vi "Butterfly_PullDown RCV_TTR_AWG.vi"(0 "Semiconductor Module Context":T2, 1 "RFPins":string[](array[string]), 2 "script name":string, 3 "R Thresholds":dbl[](array[numeric]), 4 "Capacitance":bool=TRUE, 5 "error in (no error)":errorcluster, 6 "VNAs Measurement Parameters":T1, 7 "Start_v":dbl=10.0 format="%#_13g", 8 "C_TH_Delta":dbl=2.0, 9 "Stop_v":dbl=41.0 format="%#_13g", 11 "Step_v":dbl=1.0) -> (14 "Semiconductor Module Context Out":T2, 19 "error out":errorcluster)   [LabVIEW 2013]
uses:
  <vilib>/NI_TestStand_SemiconductorModule/NI_TestStand_Semiconductor_Module.lvlibp/PinMap/General/SemiconductorModuleContext.ctl
  VNA/VNAs Measurement Parameters.ctl
  <instrlib>/niHSDIO/niHSDIO.llb/niHSDIO_ctl Trigger Script - trigID Values (Ring).ctl
  <instrlib>/niDCPower/nidcpower.llb/niDCPower Wait For Event - Event.ctl
  <vilib>/NI_TestStand_SemiconductorModule/NI_TestStand_Semiconductor_Module.lvlibp/PinMap/DC Power/PinsToNIDCPowerSessions.vi
  <vilib>/NI_TestStand_SemiconductorModule/NI_TestStand_Semiconductor_Module.lvlibp/PinMap/General/Publish/PublishDataDoubleFunctionalTest.vi
  <vilib>/NI_TestStand_SemiconductorModule/NI_TestStand_Semiconductor_Module.lvlibp/PinMap/General/Publish/PublishDataDouble2D.vi
  <vilib>/NI_TestStand_SemiconductorModule/NI_TestStand_Semiconductor_Module.lvlibp
  VNA/Pin Map API/VNA Custom Instrument.lvlib
panel:
  in  "current level":dbl=0.01 format="%_6p"
  out "VPIs 2":dbl[](array[numeric])
  out "VRLs 2":dbl[](array[numeric])
  out "S0 steps":dbl[](array[numeric]) format="%#_3g"
  out "S1 steps":dbl[](array[numeric]) format="%#_3g"
  out "S2 steps":dbl[](array[numeric]) format="%#_3g"
  out "S3 steps":dbl[](array[numeric]) format="%#_3g"
  out "appended array":dbl[][](array[numeric]) format="%#_3g"
  out "VPIs":dbl[][](array[numeric]) format="%#_3g"
  out "VRLs":dbl[][](array[numeric]) format="%#_3g"
  out "C_Free":dbl[](array[numeric])
  out "Full R Array":dbl[][][](array[numeric])
  out "step":i32
  out "sites and pins loop iter":i32
  out "BF values":dbl[](array[numeric])
  out "BF Names":string[](array[string])
  out "R Array":dbl[](array[numeric])
  out "BFSamples":i32
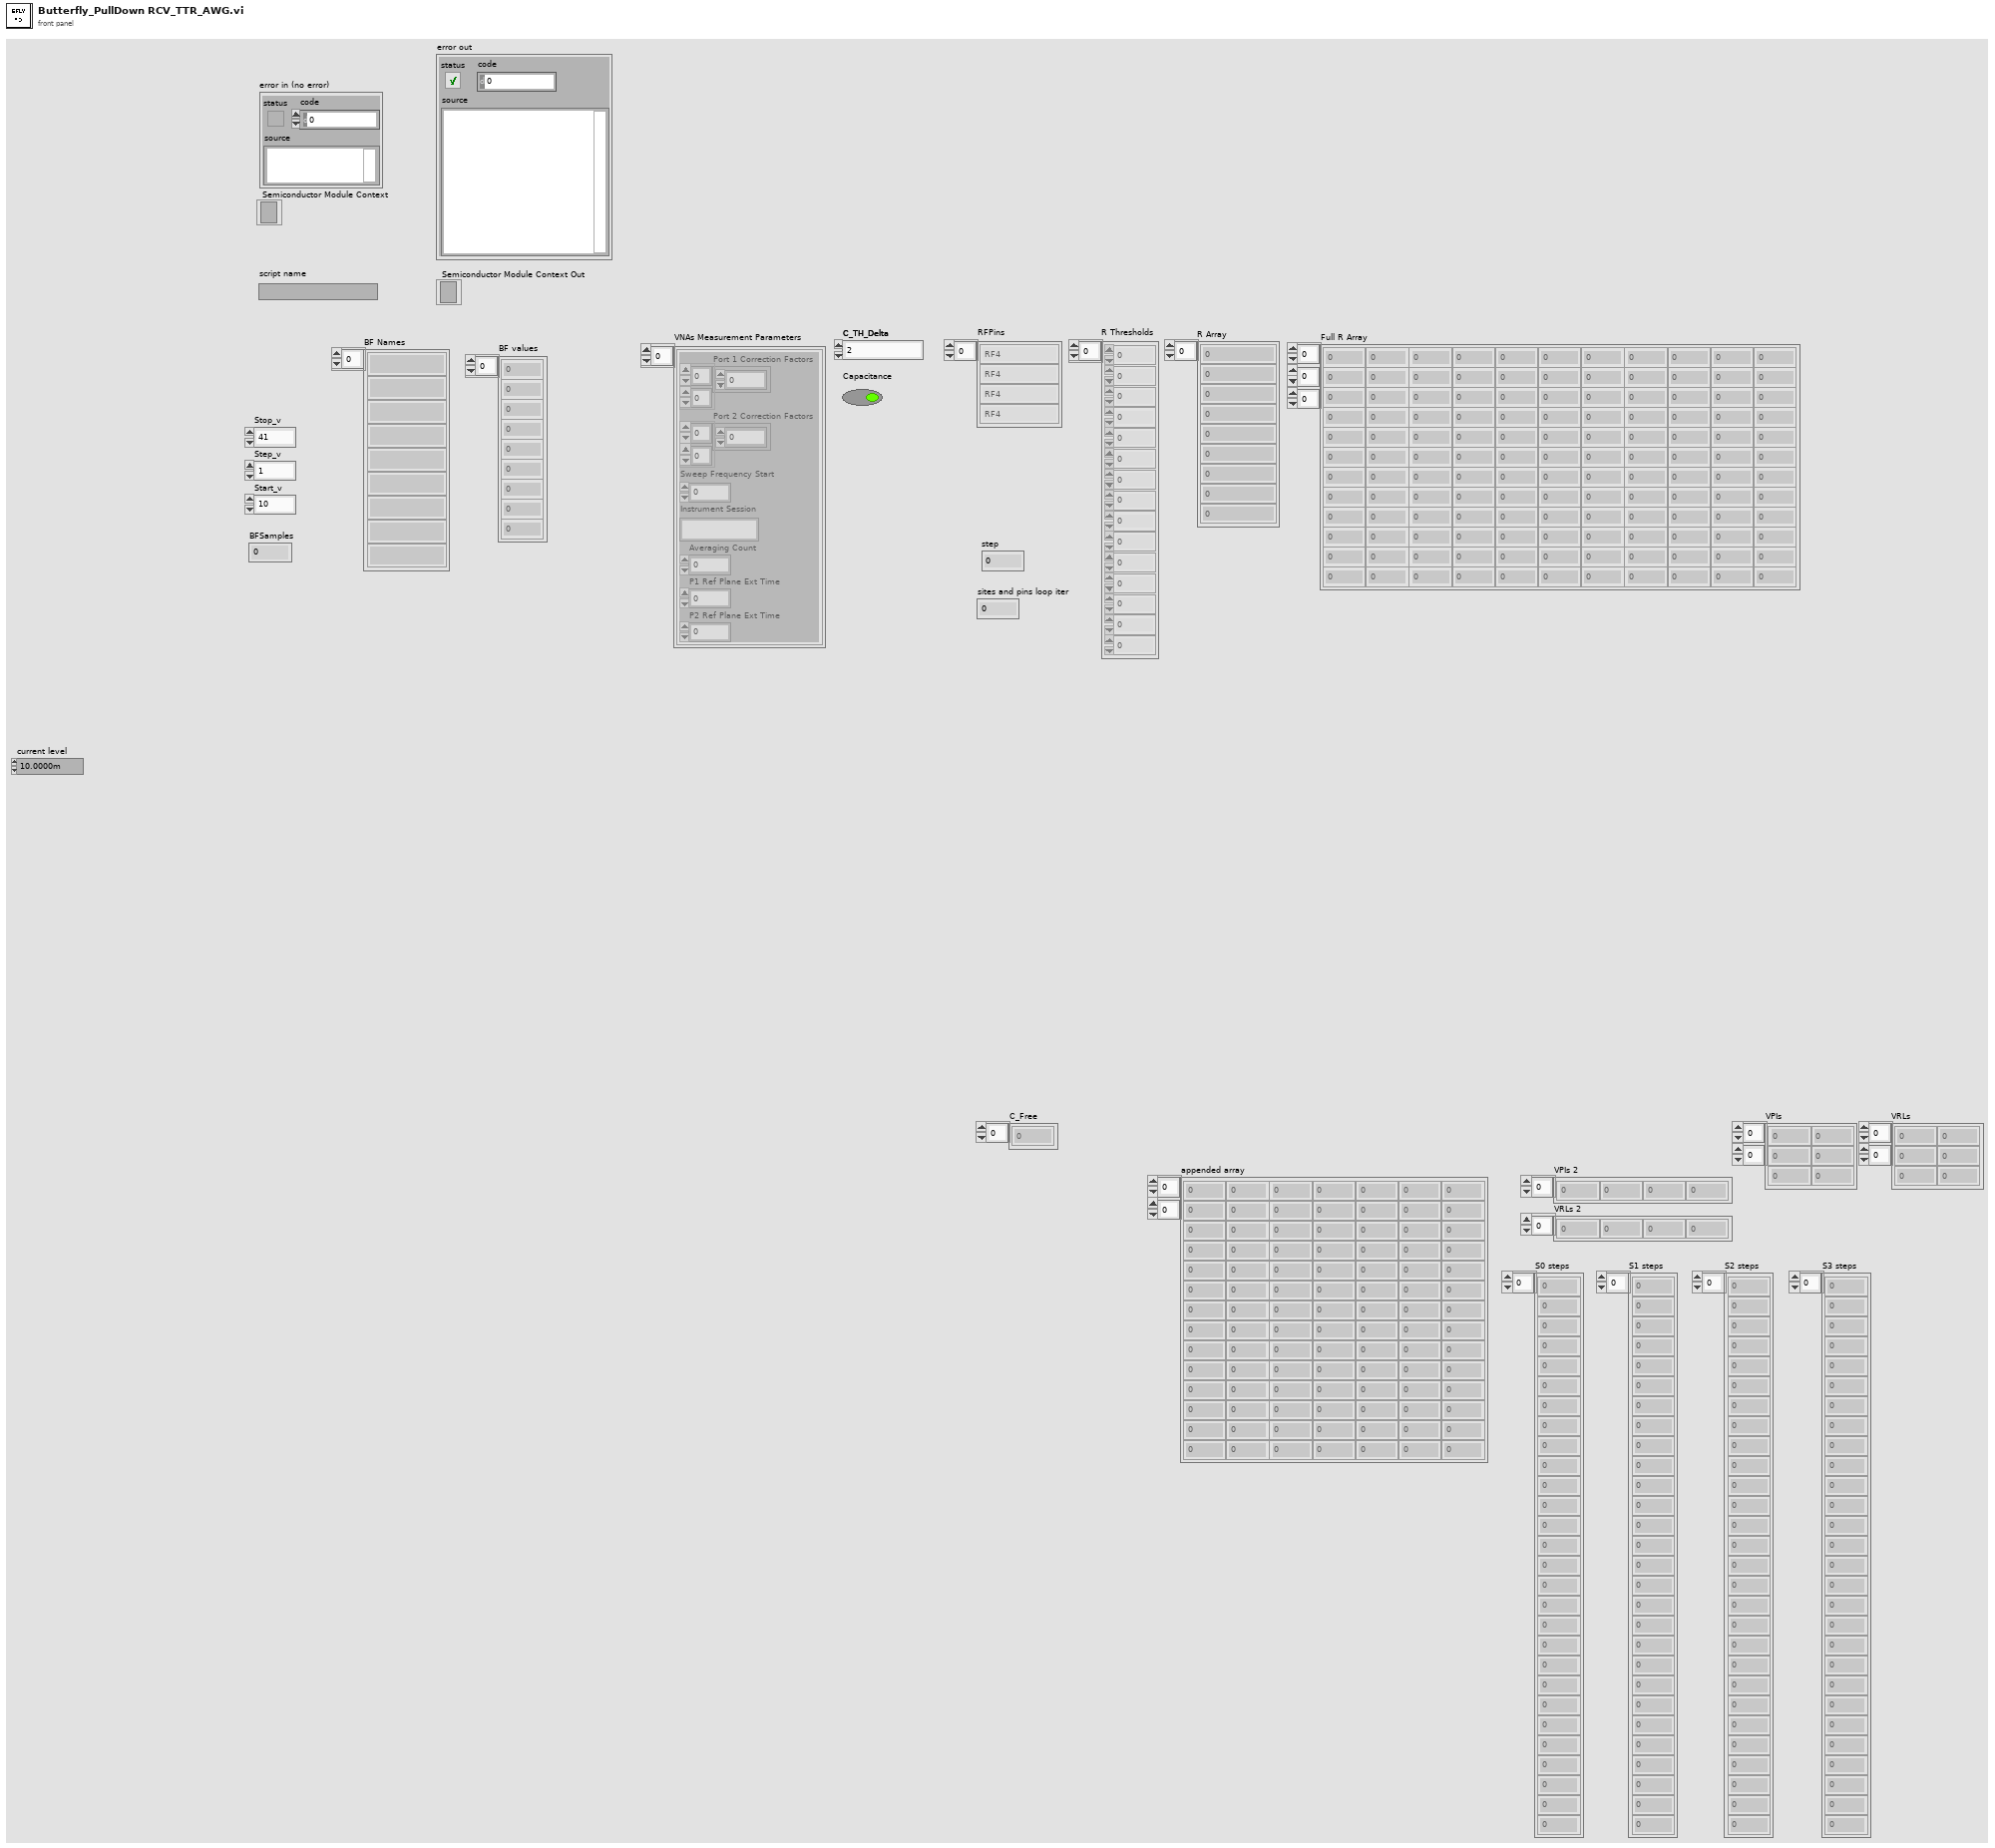
[diagram p1: front panel]
types:
  T1 = typedef "VNAs Measurement Parameters.ctl" = cluster{"Port 1 Correction Factors":cdb[][], "Port 2 Correction Factors":cdb[][], "Sweep Frequency Start":dbl, "Instrument Session":string, "Averaging Count":i32, "P1 Ref Plane Ext Time":dbl, "P2 Ref Plane Ext Time":dbl}[]
  T2 = typedef "NI_TestStand_Semiconductor_Module.lvlibp/SemiconductorModuleContext.ctl" = refnum<k7>
  T3 = typedef "niDCPower Wait For Event - Event.ctl" = i32
  T4 = typedef "niHSDIO_ctl Trigger Script - trigID Values (Ring).ctl" = string
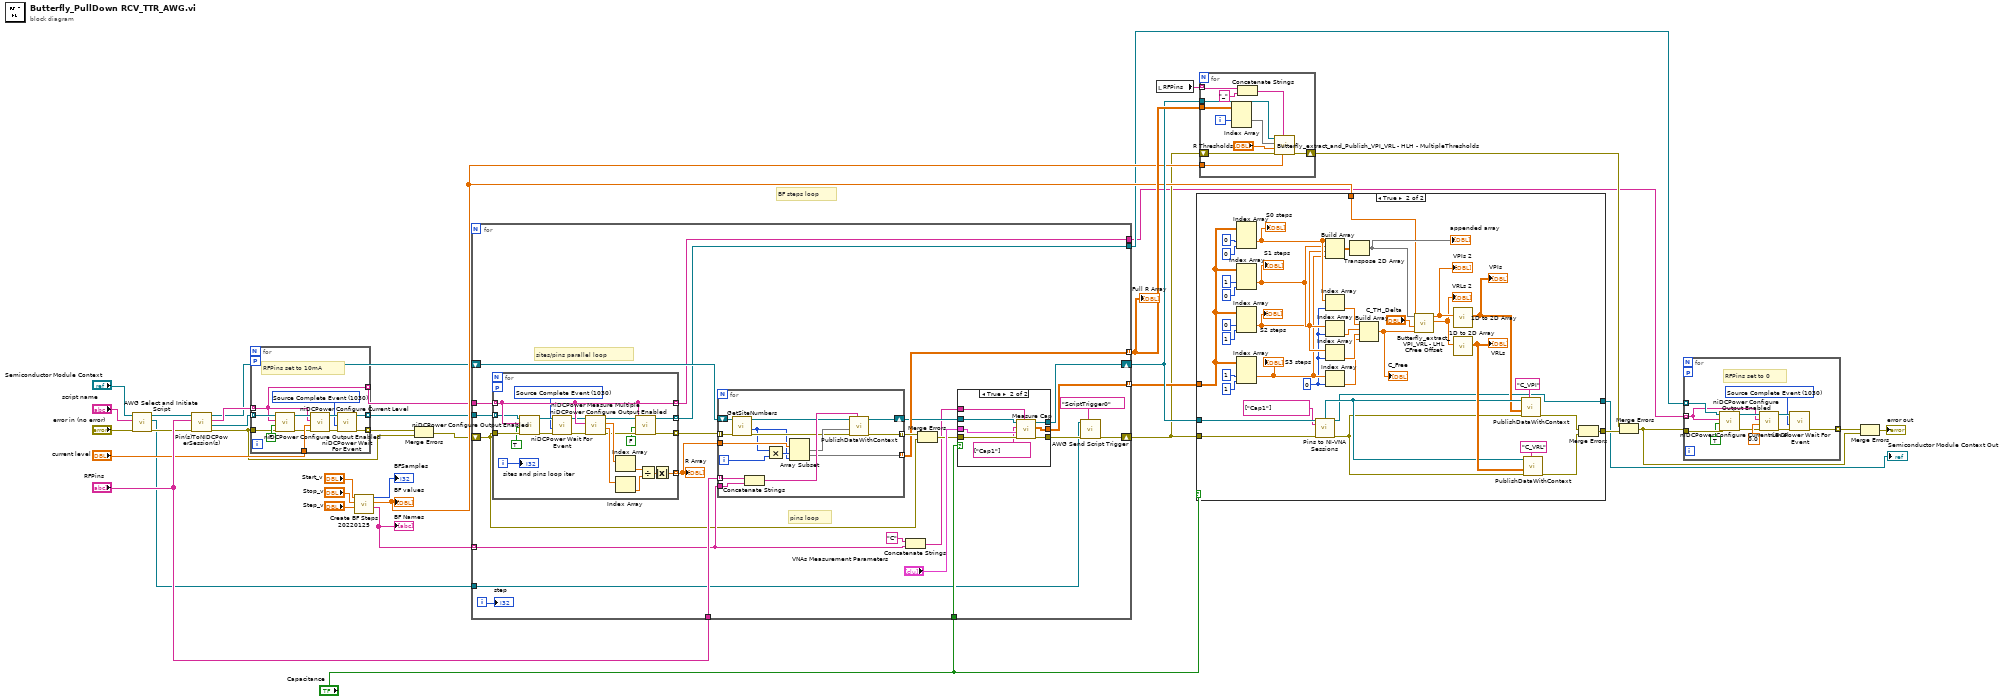
[diagram p0: block diagram]
diagram:
  # "BF steps loop"
  n1 = call "AWG Select and Initiate Script.vi"("error in (no error)"="error in (no error)", "script name"="script name", "Semiconductor Module Context"="Semiconductor Module Context") -> ("error out"=w6:errorcluster, "Sessions Out"=w1:refnum<k15>[], "Semiconductor Module Context Out"=w8:T2)  [unwired: 6 in]
  n2 = call-poly <vilib>:"Pin(s)ToNIDCPowerSession(s).vi"("error in (no error)"=w6, "Pins"="RFPins", "Semiconductor Module Context"=w8) -> ("error out"=w10:errorcluster, "Instrument Sessions"=w20:refnum<k15>[], "Channel Lists"=w19:string[], "Semiconductor Module Context Out"=w7:T2)  [unwired: 4 in, 1 out]
  n3 = for {
    tunnel: w20 -> [w43] mode=indexing
    tunnel: w19 -> [w39] mode=indexing
    tunnel: "current level" -> [w45]
    tunnel: [w38] -> w16 mode=indexing
    tunnel: [w39] -> w17 mode=indexing
    workers-P: _ -> [_]
    tunnel: w10 -> [w40]
    tunnel: [w37] -> w11 mode=indexing
    w46 = T3 1030 items=["Source Complete Event"=1030, "Measure Complete Event"=1031, "Sequence Iteration Complete Event"=1032, "Sequence Engine Done Event"=1033, "Pulse Complete Event"=1051, "Ready For Pulse Trigger Event"=1052] ("event")
    # "RFPins set to 10mA"
    n4 = call <instrlib>:"niDCPower Configure Output Enabled.vi"("error in (no error)"=w40, "output enabled"=FALSE, "channel name"=w39, "instrument handle"=w43) -> ("error out"=w41:errorcluster, "instrument handle out"=w42:refnum<k15>)  [unwired: 6 in]
    n5 = call <instrlib>:"niDCPower Configure Current Level.vi"("error in (no error)"=w41, "current level"=w45, "channel name"=w39, "instrument handle"=w42) -> ("error out"=w48:errorcluster, "instrument handle out"=w47:refnum<k15>)  [unwired: 6 in]
    n6 = call <instrlib>:"niDCPower Wait For Event.vi"("error in (no error)"=w48, "event"=w46, "instrument handle"=w47) -> ("error out"=w37:errorcluster, "instrument handle out"=w38:refnum<k15>)  [unwired: 7 in]
  }
  n7 = call "Create BF Steps 20220125.vi"("Step_v"="Step_v", "Stop_v"="Stop_v", "Start_v"="Start_v") -> ("BF Names"=w32:string[], "BF values"=w27:dbl[], "BFSamples"=→"BFSamples":i32)  [unwired: 6 in]
  "BF Names" <- w32
  "BF values" <- w27
  n8 = Merge Errors(w11, w10) -> (w5:errorcluster)
  n9 = for {
    shift-right: [w51] -> w26
    shift-left: w5 -> [w53]
    shift-right: [w60] -> w29
    shift-left: w7 -> [w58]
    tunnel: "RFPins" -> [w71]
    tunnel: w32 -> [w63] mode=indexing
    tunnel: [w69] -> w30 mode=indexing
    tunnel: "Capacitance" -> [w61]
    tunnel: [w59] -> w28 mode=indexing
    tunnel: w17 -> [w57]
    tunnel: w16 -> [w56]
    tunnel: [w55] -> w15
    tunnel: [w54] -> w14
    tunnel: w1 -> [w49]
    i -> [w73]
    # "pins loop"
    # "sites/pins parallel loop"
    n10 = for {
      tunnel: w53 -> [w111]
      tunnel: [w113] -> w70 mode=indexing
      tunnel: [w109] -> w68 mode=indexing
      workers-P: _ -> [_]
      tunnel: w57 -> [w106] mode=indexing
      tunnel: w56 -> [w105] mode=indexing
      tunnel: [w107] -> w55 mode=indexing
      tunnel: [w106] -> w54 mode=indexing
      i -> [w112]
      w98 = T3 1030 items=["Source Complete Event"=1030, "Measure Complete Event"=1031, "Sequence Iteration Complete Event"=1032, "Sequence Engine Done Event"=1033, "Pulse Complete Event"=1051, "Ready For Pulse Trigger Event"=1052] ("event")
      n11 = call <instrlib>:"niDCPower Configure Output Enabled.vi"("error in (no error)"=w111, "output enabled"=TRUE, "channel name"=w106, "instrument handle"=w105) -> ("error out"=w102:errorcluster, "instrument handle out"=w99:refnum<k15>)  [unwired: 6 in]
      n12 = call <instrlib>:"niDCPower Wait For Event.vi"("error in (no error)"=w102, "event"=w98, "instrument handle"=w99) -> ("error out"=w101:errorcluster, "instrument handle out"=w100:refnum<k15>)  [unwired: 7 in]
      n13 = call <instrlib>:"niDCPower Measure Multiple.vi"("error in (no error)"=w101, "channel name"=w106, "instrument handle"=w100) -> ("error out"=w110:errorcluster, "current measurements"=w114:dbl[], "voltage measurements"=w115:dbl[], "instrument handle out"=w108:refnum<k15>)  [unwired: 5 in]
      n14 = Index Array(array=w115) -> (element=w117:dbl)  [unwired: 1 in]
      n15 = Index Array(array=w114) -> (element=w116:dbl)  [unwired: 1 in]
      n16 = call <instrlib>:"niDCPower Configure Output Enabled.vi"("error in (no error)"=w110, "output enabled"=FALSE, "channel name"=w106, "instrument handle"=w108) -> ("error out"=w109:errorcluster, "instrument handle out"=w107:refnum<k15>)  [unwired: 6 in]
      n17 = Divide(x=w117, y=w116) -> (x/y=w118:dbl)
      n18 = Absolute Value(x=w118) -> (abs(x)=w113:dbl)
      "sites and pins loop iter" <- w112
    }
    "R Array" <- w70
    n19 = for {
      tunnel: [w92] -> w72 mode=indexing
      tunnel: w71 -> [w96] mode=indexing
      tunnel: w70 -> [w93]
      tunnel: w63 -> [w95]
      shift-right: [w90] -> w67
      shift-left: w58 -> [w87]
      tunnel: [w89] -> w69 mode=indexing
      tunnel: w68 -> [w84] mode=indexing
      i -> [w97]
      n20 = call <vilib>:"GetSiteNumbers.vi"("error in (no error)"=w84, "Semiconductor Module Context"=w87) -> ("error out"=w88:errorcluster, "Number Of Sites"=w85:i32, "Semiconductor Module Context Out"=w86:T2)  [unwired: 6 in, 1 out]
      n21 = Concatenate Strings(w96, w95) -> (w91:string)
      n22 = Multiply(x=w85, y=w97) -> (x*y=w94:i32)
      n23 = Array Subset(array=w93, index=w94, length=w85) -> (w89:dbl[])
      n24 = call-poly <vilib>:"PublishDataWithContext.vi"("Published Data Id"=w91, "error in (no error)"=w88, "Data In"=w89, "Semiconductor Module Context"=w86) -> ("error out"=w92:errorcluster, "Semiconductor Module Context Out"=w90:T2)  [unwired: 6 in]
    }
    n25 = Concatenate Strings("C" ("string"), w63) -> (w62:string)
    n26 = Merge Errors(w72, w53) -> (w65:errorcluster)
    n27 = case shown="True" w61 {
      tunnel: w67 -> [w75 w83]
      tunnel: [w75 w82] -> w60
      tunnel: [w74 w80] -> w52
      tunnel: w62 -> [_ w76]
      tunnel: "VNAs Measurement Parameters" -> [_ w78]
      tunnel: [_ w79] -> w59
      tunnel: w65 -> [w74 w81]
      frame False {
      }
      frame True {
        n28 = call "Measure Cap.vi"("Measurement Id"=w76, "error in (no error)"=w81, "VNAs Measurement Parameters"=w78, "Pins"=string[] ["Cap1"] ("Capacitance Pins"), "Semiconductor Module Context"=w83) -> ("error out"=w80:errorcluster, "Multisite Cap Data"=w79:dbl[][], "Semiconductor Module Context Out"=w82:T2)  [unwired: 4 in]
      }
    }
    n29 = call "AWG Send Script Trigger.vi"("trigger id (script trigger 0)"=T4 "ScriptTrigger0", "error in (no error)"=w52, "AWG Sessions In"=w49) -> ("error out"=w51:errorcluster)  [unwired: 7 in, 1 out]
    "step" <- w73
  }
  "Full R Array" <- w30
  n30 = local read "RFPins"() -> (w31:string[])
  n31 = case shown="True" "Capacitance" {
    tunnel: [w119 w139] -> w22
    tunnel: [w120 w157] -> w23
    tunnel: w29 -> [w119 w156]
    tunnel: w26 -> [w120 w152]
    tunnel: w27 -> [_ w124]
    tunnel: w28 -> [_ w143]
    frame False {
    }
    frame True {
      w132 = 0 ("index")
      n32 = Index Array(array=w143, index (dim 1)=0 ("disabled index (row)"), index (dim 2)=0 ("disabled index (col)")) -> (element=w136:dbl[])  [unwired: 1 in]
      "S0 steps" <- w136
      n33 = Index Array(array=w143, index (dim 1)=1 ("index (row)"), index (dim 2)=0 ("index (col)")) -> (element=w135:dbl[])  [unwired: 1 in]
      "S1 steps" <- w135
      n34 = Index Array(array=w143, index (dim 1)=0 ("index (row)"), index (dim 2)=1 ("index (col)")) -> (element=w134:dbl[])  [unwired: 1 in]
      "S2 steps" <- w134
      n35 = Index Array(array=w143, index (dim 1)=1 ("index (row)"), index (dim 2)=1 ("index (col)")) -> (element=w133:dbl[])  [unwired: 1 in]
      "S3 steps" <- w133
      n36 = call "Pins to NI-VNA Sessions.vi"("Semiconductor Module Context"=w156, "Pins"=string[] ["Cap1"] ("Capacitance Pins"), "error in (no error)"=w152) -> ("Pin Query Context"=w142:refnum<class "MultiplePinMultipleSessionQueryContext.lvclass">, "Semiconductor Module Context Out"=w139:T2, "error out"=w137:errorcluster)  [unwired: 8 in, 2 out]
      n37 = Build Array(w136, w135, w134, w133) -> (w127:dbl[][])
      n38 = Index Array(array=w136, index=w132) -> (element=w131:dbl)
      n39 = Index Array(array=w135, index=w132) -> (element=w130:dbl)
      n40 = Index Array(array=w134, index=w132) -> (element=w129:dbl)
      n41 = Index Array(array=w133, index=w132) -> (element=w128:dbl)
      n42 = Transpose 2D Array(2D array=w127) -> (transposed array=w125:dbl[][])
      "appended array" <- w125
      n43 = Build Array(w131, w130, w129, w128) -> (w126:dbl[])
      "C_Free" <- w126
      n44 = call "Butterfly_extract_VPI_VRL - LHL CFree Offset.vi"("C_Free"=w126, "Delta"="C_TH_Delta", "Voltage Array"=w124, "Result Array In"=w125) -> ("VRLs"=w121:dbl[], "VPIs"=w122:dbl[])  [unwired: 6 in]
      "VPIs 2" <- w122
      "VRLs 2" <- w121
      n45 = call "1D to 2D Array.vi"("1D Array"=w122) -> ("2D Array"=w141:dbl[][])  [unwired: 10 in]
      "VPIs" <- w141
      n46 = call "1D to 2D Array.vi"("1D Array"=w121) -> ("2D Array"=w155:dbl[][])  [unwired: 10 in]
      "VRLs" <- w155
      n47 = call-poly <vilib>:"PublishDataWithContext.vi"("Published Data Id"="C_VPI", "error in (no error)"=w137, "Data In"=w141, "Pin Query Context"=w142) -> ("error out"=w138:errorcluster)  [unwired: 6 in, 1 out]
      n48 = call-poly <vilib>:"PublishDataWithContext.vi"("Published Data Id"="C_VRL", "error in (no error)"=w137, "Data In"=w155, "Pin Query Context"=w142) -> ("error out"=w158:errorcluster)  [unwired: 6 in, 1 out]
      n49 = Merge Errors(w138, w158) -> (w157:errorcluster)
    }
  }
  "Semiconductor Module Context Out" <- w22
  n50 = for {
    tunnel: w31 -> [w163] mode=indexing
    tunnel: w30 -> [w168]
    shift-right: [w164] -> w24
    shift-left: w26 -> [w165]
    tunnel: w29 -> [w160]
    tunnel: w27 -> [w159]
    i -> [w169]
    n51 = Index Array(array=w168, index (dim 1)=w169) -> (element=w166:dbl[][])  [unwired: 2 in]
    n52 = Concatenate Strings(w163, "_" ("string")) -> (w161:string)
    n53 = call "Butterfly_extract_and_Publish_VPI_VRL - HLH - MultipleThresholds.vi"("Voltages Array"=w159, "ID Prefix"=w161, "error in (no error)"=w165, "Thresholds"="R Thresholds", "Result Array In"=w166, "Semiconductor Module Context"=w160) -> ("error out"=w164:errorcluster)  [unwired: 5 in]
  }
  n54 = Merge Errors(w24, w23) -> (w2:errorcluster)
  n55 = for {
    tunnel: w15 -> [w173] mode=indexing
    tunnel: w14 -> [w171] mode=indexing
    workers-P: _ -> [_]
    tunnel: w2 -> [w175]
    tunnel: [w177] -> w13 mode=indexing
    w176 = T3 1030 items=["Source Complete Event"=1030, "Measure Complete Event"=1031, "Sequence Iteration Complete Event"=1032, "Sequence Engine Done Event"=1033, "Pulse Complete Event"=1051, "Ready For Pulse Trigger Event"=1052] ("event")
    # "RFPins set to 0"
    n56 = call <instrlib>:"niDCPower Configure Output Enabled.vi"("error in (no error)"=w175, "output enabled"=TRUE, "channel name"=w171, "instrument handle"=w173) -> ("error out"=w174:errorcluster, "instrument handle out"=w172:refnum<k15>)  [unwired: 6 in]
    n57 = call <instrlib>:"niDCPower Configure Current Level.vi"("error in (no error)"=w174, "current level"=0.0, "channel name"=w171, "instrument handle"=w172) -> ("error out"=w180:errorcluster, "instrument handle out"=w179:refnum<k15>)  [unwired: 6 in]
    n58 = call <instrlib>:"niDCPower Wait For Event.vi"("error in (no error)"=w180, "event"=w176, "instrument handle"=w179) -> ("error out"=w177:errorcluster)  [unwired: 7 in, 1 out]
  }
  n59 = Merge Errors(w13, w2) -> (→"error out":errorcluster)
